vi "Create MetaData Element.vi"(6 "MetaData Parameters":T4, 7 "Channel Properties":T3, 8 "error in (no error)":errorcluster, 9 "Type":T1, 10 "Name":string, 11 "Refnum In":T2 format="%.0x") -> (0 "error out":errorcluster, 2 "Channel Refnum":T2 format="%.0x", 3 "Refnum Out":T2 format="%.0x")   [LabVIEW 2018, in "Instrument Addon Scripting API.lvlib"]
uses:
  Instrument Addon Scripting API.lvlib
  Addon/Addon Shared/Types/MetaData Parameters.ctl
  Addon/Addon Shared/Types/Protocol Data Type.ctl
  Addon/Addon Shared/Types/Metadata Channel Type.ctl
  Addon/Addon Shared/Types/Type Cast Type.ctl
  Addon/Addon Shared/Types/Endian.ctl
  <vilib>/NI Veristand/Custom Device API/Custom Device Item Ref.ctl
  TypeDefs/Channel Properties.ctl
  TypeDefs/MetaData Type.ctl
  <vilib>/NI Veristand/Custom Device API/Custom Device Channel.ctl
  <vilib>/NI Veristand/Custom Device API/Custom Device Channel Type.ctl
  Addon/Addon Shared/Types/FG Control.ctl
  Addon/Addon Shared/SubVIs/Constants.vi
  <vilib>/NI Veristand/Custom Device Tools/Custom Device Utility Library/NI VeriStand - Search for Item by GUID.vi
  <vilib>/NI Veristand/Custom Device API/NI VeriStand - Get Item Property.vi
  <vilib>/NI Veristand/Custom Device API/Get Item Property (U32).vi
  <vilib>/NI Veristand/Custom Device API/Get Item Property (String Array).vi
  <vilib>/NI Veristand/Custom Device API/Get Item Property (String).vi
  <vilib>/NI Veristand/Custom Device API/NI VeriStand - Set Item Property.vi
  <vilib>/NI Veristand/Custom Device API/Set Item Property (U32).vi
  <vilib>/NI Veristand/Custom Device API/Set Item Property (String Array).vi
  <vilib>/NI Veristand/Custom Device API/NI VeriStand - Get Item Children.vi
  Addon/Addon Shared/SubVIs/Set Channel Value Table.vi
  <vilib>/NI Veristand/Custom Device API/Set Item Property (String).vi
  <vilib>/NI Veristand/Custom Device Tools/Custom Device Utility Library/Custom Device Utility Library.lvlib
  Addon/Addon Shared/Instrument Addon Shared.lvlib
  <vilib>/NI Veristand/Custom Device API/Custom Device API.lvlib
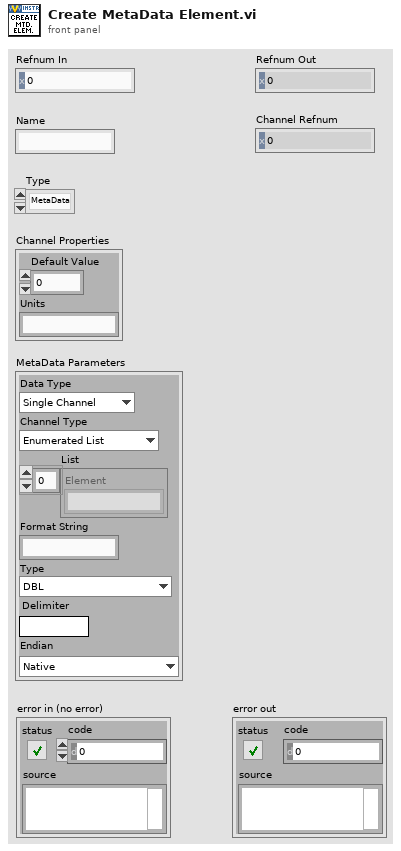
[diagram p1: front panel]
types:
  T1 = typedef "Instrument Addon Scripting API.lvlib/MetaData Type.ctl" = enum16{"MetaData", "Global MetaData"}
  T2 = typedef "Custom Device API.lvlib/Custom Device Item Ref.ctl" = u64
  T3 = typedef "Channel Properties.ctl" = cluster{"Default Value":dbl, "Units":string}
  T4 = typedef "Instrument Addon Shared.lvlib/MetaData Parameters.ctl" = cluster{"Data Type":T5, "Channel Type":T6, "List":string[], "Format String":string, "Type":T7, "Delimiter":string, "Endian":T8}
  T5 = typedef "Instrument Addon Shared.lvlib/Protocol Data Type.ctl" = enum16{"Single Channel", "Array"}
  T6 = typedef "Instrument Addon Shared.lvlib/Metadata Channel Type.ctl" = enum16{"Enumerated List", "Format", "Type Cast"}
  T7 = typedef "Instrument Addon Shared.lvlib/Type Cast Type.ctl" = enum16{"DBL", "SGL", "U64", "U32", "U16", "U8", "I64", "I32", "I16", "I8"}
  T8 = typedef "Instrument Addon Shared.lvlib/Endian.ctl" = enum16{"Native", "Little", "Big"}
  T9 = typedef "Custom Device API.lvlib/Custom Device Channel Type.ctl" = enum16{"Input", "Output"}
  T10 = typedef "Instrument Addon Shared.lvlib/FG Control.ctl" = enum16{"Get", "Set"}
  T11 = typedef "Custom Device API.lvlib/Custom Device Channel.ctl" = cluster{"Type":T9, "Units":string, "Default Value":dbl, "Faultable":bool, "Scalable":bool}
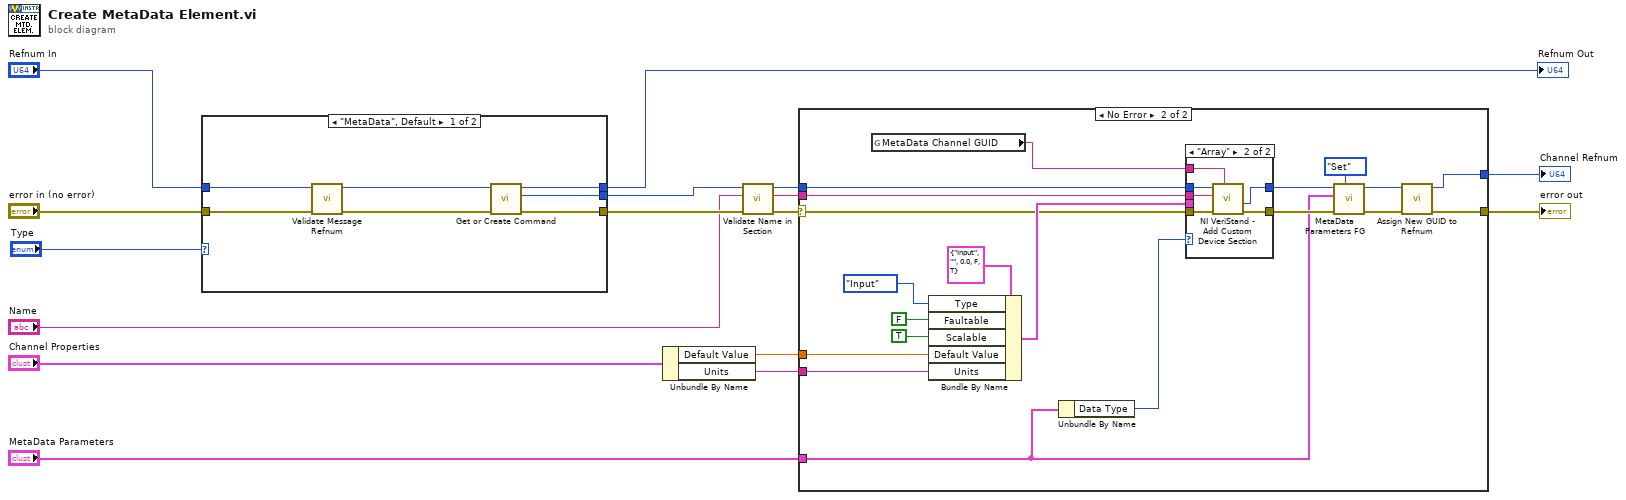
[diagram p0: block diagram]
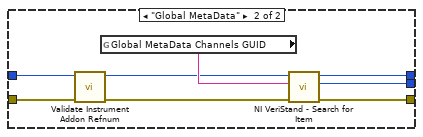
[diagram p2: hidden frame]
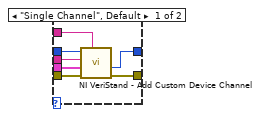
[diagram p4: hidden frame]
diagram:
  n1 = case shown="\"MetaData\", Default" "Type" {
    tunnel: [w21 w31] -> w1
    tunnel: [w23 w30] -> w6
    tunnel: "error in (no error)" -> [w19 w26]
    tunnel: "Refnum In" -> [w20 w27]
    tunnel: [w22 w28] -> w8
    frame "MetaData", Default {
      n2 = call "Validate Message Refnum.vi"("error in (no error)"=w19, "Message in"=w20) -> ("error out"=w17:errorcluster, "Message out"=w18:T2)  [unwired: 8 in]
      n3 = call "Get or Create Command.vi"("error in (no error)"=w17, "Message Refnum In"=w18) -> ("error out"=w23:errorcluster, "Command Refnum"=w21:T2, "Message Refnum Out"=w22:T2)  [unwired: 7 in]
    }
    frame "Global MetaData" {
      n4 = call "Validate Instrument Addon Refnum.vi"("Error In"=w26, "Refnum In"=w27) -> ("Error Out"=w25:errorcluster, "Refnum Out"=w24:T2)  [unwired: 7 in, 1 out]
      n5 = global read "Constants.vi" "Global MetaData Channels GUID"() -> (w29:string)
      n6 = call-poly <vilib>:"NI VeriStand - Search for Item.vi"("error in"=w25, "Item GUID"=w29, "Section Ref in"=w24) -> ("error out"=w30:errorcluster, "Item Ref"=w31:T2, "Section Ref out"=w28:T2)  [unwired: 5 in, 1 out]
    }
  }
  "Refnum Out" <- w8
  n7 = Unbundle By Name("Channel Properties") -> ("Default Value"=w11:dbl, "Units"=w10:string)
  n8 = call "Validate Name in Section.vi"("error in (no error)"=w6, "Name In"="Name", "Refnum In"=w1) -> ("error out"=w3:errorcluster, "Name Out"=w4:string, "Refnum Out"=w5:T2)  [unwired: 6 in]
  n9 = case shown="No Error" w3 {
    selector: w3 -> [w32 w34]
    tunnel: w5 -> [w33 w53]
    tunnel: w4 -> [_ w52]
    tunnel: [w32 w47] -> w14
    tunnel: [w33 w45] -> w15
    tunnel: "MetaData Parameters" -> [_ w37]
    tunnel: w11 -> [_ w39]
    tunnel: w10 -> [_ w38]
    frame Error {
      # "Error case - Label is already in use"
    }
    frame No Error {
      n10 = global read "Constants.vi" "MetaData Channel GUID"() -> (w35:string)
      n11 = Bundle By Name(cluster=T11 {"Type"=enum."Input", "Units"="", "Default Value"=0.0, "Faultable"=FALSE, "Scalable"=TRUE} ("Channel"), "Type"=Custom_Device_Channel_Type."Input", "Faultable"=FALSE, "Scalable"=TRUE, "Default Value"=w39, "Units"=w38) -> (w40:T11)
      n12 = Unbundle By Name(w37) -> ("Data Type"=w36:T5)
      n13 = case shown="\"Array\"" w36 {
        tunnel: w35 -> [w55 w62]
        tunnel: w53 -> [w60 w63]
        tunnel: w52 -> [w59 w61]
        tunnel: w34 -> [w58 w66]
        tunnel: [w57 w65] -> w50
        tunnel: [w54 w64] -> w49
        tunnel: w40 -> [w56 _]
        frame "Single Channel", Default {
          n14 = call <vilib>:"NI VeriStand - Add Custom Device Channel.vi"("GUID (Default Channel)"=w55, "error in (no error)"=w58, "Channel"=w56, "Channel Name"=w59, "Parent Ref in"=w60) -> ("error out"=w57:errorcluster, "Channel Ref"=w54:T2)  [unwired: 3 in, 2 out]
        }
        frame "Array" {
          n15 = call <vilib>:"NI VeriStand - Add Custom Device Section.vi"("GUID (Default Section)"=w62, "error in (no error)"=w66, "Section Name"=w61, "Parent Ref in"=w63) -> ("error out"=w65:errorcluster, "Section Ptr"=w64:T2)  [unwired: 4 in, 2 out]
        }
      }
      n16 = call "MetaData Parameters FG.vi"("Action"=FG_Control."Set", "error in (no error)"=w50, "MetaData Parameters"=w37, "Item Ref in"=w49) -> ("error out"=w48:errorcluster, "Item Ref out"=w46:T2)  [unwired: 5 in, 1 out]
      n17 = call "Assign New GUID to Refnum.vi"("error in (no error)"=w48, "Item Ref in"=w46) -> ("error out"=w47:errorcluster, "Item Ref out"=w45:T2)  [unwired: 8 in]
    }
  }
  "Channel Refnum" <- w15
  "error out" <- w14
